vi "Actions.vi"(2 "direction":T1(ring), 3 "X coordinate IN":i32, 4 "Y coordinate IN":i32) -> (0 "X coordinate OUT":i32, 1 "Y coordinate OUT":i32)   [LabVIEW 2014]
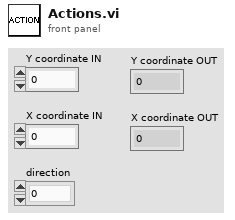
[diagram p1: front panel]
types:
  T1 = enum16{"0", "1", "2", "3", "4", "5", "6", "7", "8", "9", "A", "B", "C", "D", "E", "F", "G", "H", "I", "J", "K", "L", "M", "N", "O", "P", "Q", "R", "S", "T", "U", "V", "W", "X", "Y", "Z", "F1", "F2", "F3", "F4", "F5", "F6", "F7", "F8", "F9", "F10", "F11", "F12", "F13", "F14", "F15", "ADD", "BACK", "BACKSLASH", "CAPITAL", "COMMA", "DECIMAL", "DELETE", "DIVIDE", "DOWN", "END", "EQUALS", "ESCAPE", "GRAVE (`)", "HOME", "INSERT", "LBRACKET", "LCONTROL", "LEFT", "L ALT", "LSHIFT", "LWIN", "MINUS", "MULTIPLY", "NEXT", "NUMLOCK", "NUMPAD_0", "NUMPAD_1", "NUMPAD_2", "NUMPAD_3", "NUMPAD_4", "NUMPAD_5", "NUMPAD_6", "NUMPAD_7", "NUMPAD_8", "NUMPAD_9", "PAUSE", "PERIOD", "PRIOR (PG UP)", "RBRACKET", "RCONTROL", "RETURN", "RIGHT", "R ALT", "RSHIFT", "RWIN", "SCROLL", "SEMICOLON", "SLASH", "SPACE", "SUBTRACT", "TAB", "UP", "ENTER (num pad)", "' (quote)"}
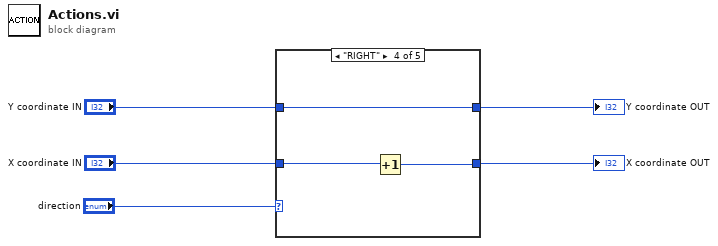
[diagram p0: block diagram]
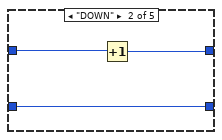
[diagram p3: hidden frame]
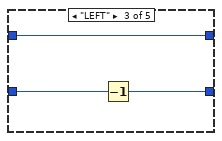
[diagram p4: hidden frame]
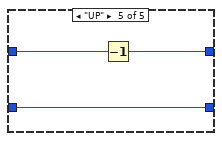
[diagram p5: hidden frame]
diagram:
  n1 = case shown="\"RIGHT\"" "direction" {
    tunnel: "X coordinate IN" -> [w6 w8 w13 w16 w17]
    tunnel: "Y coordinate IN" -> [w7 w10 w11 w14 w19]
    tunnel: [w7 w9 w11 w14 w18] -> w4
    tunnel: [w6 w8 w12 w15 w17] -> w5
    frame "0", Default {
    }
    frame "DOWN" {
      n2 = Increment(x=w10) -> (x+1=w9:i32)
    }
    frame "LEFT" {
      n3 = Decrement(x=w13) -> (x-1=w12:i32)
    }
    frame "RIGHT" {
      n4 = Increment(x=w16) -> (x+1=w15:i32)
    }
    frame "UP" {
      n5 = Decrement(x=w19) -> (x-1=w18:i32)
    }
  }
  "X coordinate OUT" <- w5
  "Y coordinate OUT" <- w4
